vi "OpenCVCam_LiveCapture.vi"(8 "error in (no error)":errorcluster, 10 "Cmd Data":variant, 11 "OpenCVCam in":refnum<class>) -> (0 "error out":errorcluster, 2 "Reply Data":variant, 3 "OpenCVCam out":refnum<class>, 4 "Exit":bool)   [LabVIEW 2021, in "OpenCVCam.lvclass"]
uses:
  OpenCVCam.lvclass
  OpenCVCam.lvclass/OpenCVCam.ctl
  OpenCVCam_UiCallBackEvents.ctl
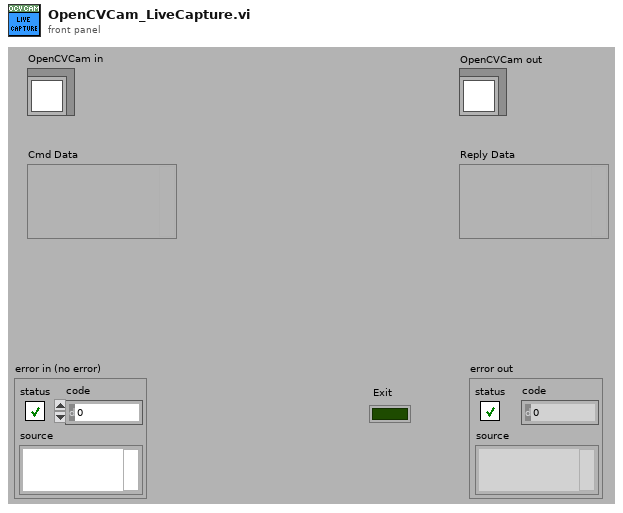
[diagram p1: front panel]
types:
  T1 = typedef "OpenCVCam.lvclass/OpenCVCam_UiCallBackEvents.ctl" = enum16{"Default", "PersistentDataUpdated", "NewPicture", "Worker 1: Do Something"}
  T2 = typedef "OpenCVCam.lvclass/State.ctl" = enum16{"Idle", "Initialized", "Acquiring"}
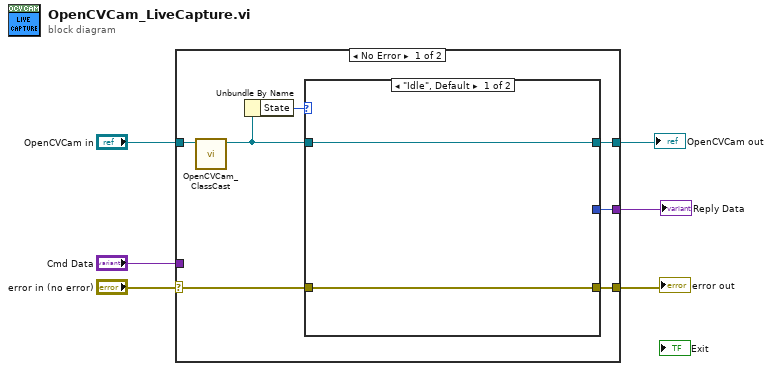
[diagram p0: block diagram]
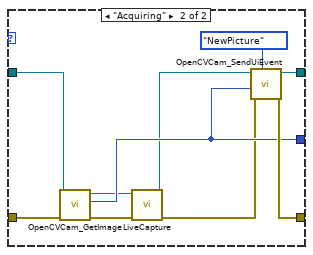
[diagram p2: hidden frame]
diagram:
  n1 = case shown="No Error" "error in (no error)" {
    selector: "error in (no error)" -> [w9 w28]
    tunnel: [w11 w28] -> w5
    tunnel: [w10 w27] -> w3
    tunnel: "Cmd Data" -> [_ w27]
    tunnel: "OpenCVCam in" -> [w13 w26]
    tunnel: [w12 w26] -> w1
    frame No Error {
      n2 = call "OpenCVCam_ClassCast.vi"("OpenCVCam in"=w13) -> ("OpenCVCam out"=w8:refnum<class "OpenCVCam.lvclass">)  [unwired: 10 in]
      n3 = Unbundle By Name(w8) -> ("State"=w7:T2)
      n4 = case shown="\"Idle\", Default" w7 {
        tunnel: [w15 w25] -> w12
        tunnel: [w14 w24] -> w11
        tunnel: [_ w23] -> w10
        tunnel: w9 -> [w14 w21]
        tunnel: w8 -> [w15 w19]
        frame "Idle", Default {
        }
        frame "Acquiring" {
          n5 = call "OpenCVCam_GetImage.vi"("error in (no error)"=w21, "OpenCVCam in"=w19) -> ("error out"=w20:errorcluster, "new picture"=w23:picture, "OpenCVCam out"=w17:refnum<class "OpenCVCam.lvclass">)  [unwired: 7 in]
          n6 = call-dynamic "LiveCapture.vi"("error in (no error)"=w20, "OpenCVCam in"=w17) -> ("error out"=w18:errorcluster, "OpenCVCam out"=w16:refnum<class "OpenCVCam.lvclass">)  [unwired: 8 in]
          n7 = call "OpenCVCam_SendUiEvent.vi"("UiEventNames"=OpenCVCam_UiCallBackEvents."NewPicture", "ErrorIn"=w18, "Data"=w23, "OpenCVCam in"=w16) -> ("ErrorOut"=w24:errorcluster, "OpenCVCam out"=w25:refnum<class "OpenCVCam.lvclass">)  [unwired: 6 in]
        }
      }
    }
    frame Error {
    }
  }
  "error out" <- w5
  "OpenCVCam out" <- w1
  "Reply Data" <- w3
